vi "BuildMsg.vi"(8 "error in (no error)":errorcluster, 10 "Msg to be build":string, 11 "CS++Actor in":refnum<class "CS++Actor.lvclass">) -> (0 "error out":errorcluster, 3 "CS++Actor out":refnum<class "CS++Actor.lvclass">)   [LabVIEW 2014, in "CS++Actor.lvlib" / "CS++Actor.lvclass"]
doc: "Build Msg Command."
uses:
  CS++Actor.lvclass
  CSPP_Message/CS++Message.lvclass
  CS++Actor.lvclass/CS++Actor.ctl
  CSPP_Message/CS++Message.lvclass/CS++Message.ctl
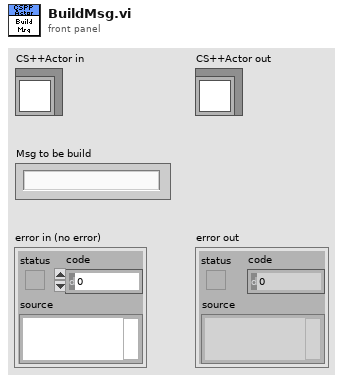
[diagram p1: front panel]
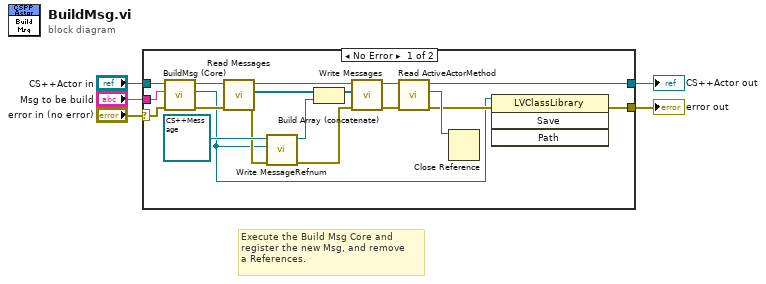
[diagram p0: block diagram]
diagram:
  # "Execute the Build Msg Core and \nregister the new Msg, and remove \na References."
  n1 = case shown="No Error" "error in (no error)" {
    selector: "error in (no error)" -> [w16 w26]
    tunnel: [w6 w26] -> w4
    tunnel: [w8 w25] -> w2
    tunnel: "CS++Actor in" -> [w17 w25]
    tunnel: "Msg to be build" -> [w13 _]
    frame No Error {
      n2 = call-dynamic "BuildMsg (Core).vi"("error in (no error)"=w16, "Msg to be build"=w13, "CS++Actor in"=w17) -> ("error out"=w15:errorcluster, "ActiveMessageClass"=w7:refnum<vi>, "CS++Actor out"=w14:refnum<class "CS++Actor.lvclass">)  [unwired: 6 in]
      n3 = call "Read Messages.vi"("error in (no error)"=w15, "CS++Actor in"=w14) -> ("error out"=w19:errorcluster, "Messages"=w23:refnum<class "CS++Message.lvclass">[], "CS++Actor out"=w24:refnum<class "CS++Actor.lvclass">)  [unwired: 7 in]
      n4 = call "Write MessageRefnum.vi"("error in (no error)"=w19, "MessageRefnum"=w7, "CS++Message in"=refnum<class "CS++Message.lvclass"> refnum ("CS++Message.lvlib:CS++Message.lvclass")) -> ("error out"=w18:errorcluster, "CS++Message out"=w20:refnum<class "CS++Message.lvclass">)  [unwired: 7 in]
      n5 = Build Array (concatenate)(w23, w20) -> (w22:refnum<class "CS++Message.lvclass">[])
      n6 = call "Write Messages.vi"("error in (no error)"=w18, "Messages"=w22, "CS++Actor in"=w24) -> ("error out"=w11:errorcluster, "CS++Actor out"=w12:refnum<class "CS++Actor.lvclass">)  [unwired: 7 in]
      n7 = call "Read ActiveActorMethod.vi"("error in (no error)"=w11, "CS++Actor in"=w12) -> ("error out"=w9:errorcluster, "ActiveActorMethod"=w10:refnum<vi>, "CS++Actor out"=w8:refnum<class "CS++Actor.lvclass">)  [unwired: 7 in]
      n8 = Close Reference(reference=w10) -> ()  [unwired: 1 in, 1 out]
      n9 = invoke class="LVClassLibrary" method="Save"(reference=w7, error in=w9) -> (error out=w6:errorcluster)  [unwired: 2 in, 3 out]
    }
    frame Error {
    }
  }
  "error out" <- w4
  "CS++Actor out" <- w2
